vi "WPI_SimpleGyro_Loop.vi"(8 "error in":errorcluster, 11 "SimpleGyroDevRef":T1) -> (0 "error out":errorcluster)   [LabVIEW 2014, in "SimpleGyro.lvlib"]
doc: "Periodically reads the SimpleGyro and makes data available to your robot project. Place this block within PeriodicTasks.vi."
uses:
  SimpleGyro.lvlib
  WPI_SimpleGyroDevRef.ctl
  <vilib>/Rock Robotics/SystemInterfaces/Typedef/FPGA_TypedefDigitalModule.ctl
  <vilib>/Rock Robotics/SystemInterfaces/spilib/spi_bus.ctl
  <vilib>/Rock Robotics/WPI/SPI/WPI_SPIDevRef.ctl
  <vilib>/Platform/TimedLoop/XDataNode/timing_clust.ctl
  <vilib>/Platform/TimedLoop/XDataNode/nitl_modes.ctl
  <vilib>/Platform/TimedLoop/XDataNode/wakeup.ctl
  <vilib>/platform/TimedLoop/XDataNode/XDataNode.xnode
  <vilib>/Platform/TimedLoop/XDataNode/XDNodeRunTimeDep.lvlib
  <vilib>/ptbypt/NI_PtbyPt.lvlib
panel:
  out "mean":dbl format="%0.2f"
  in  "Calibrate":bool
  out "Angle":dbl
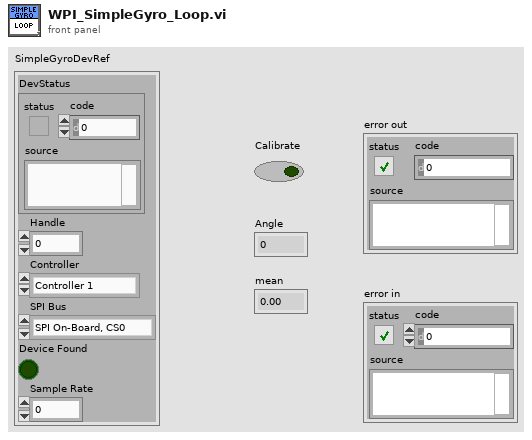
[diagram p1: front panel]
types:
  T1 = typedef "SimpleGyro.lvlib/WPI_SimpleGyroDevRef.ctl" = cluster{"DevStatus":errorcluster, "Handle":i32, "Controller":T2, "SPI Bus":T3, "Device Found":bool, "Sample Rate":dbl}
  T2 = typedef "FPGA_TypedefDigitalModule.ctl" = enum16{"Controller 1"}
  T3 = typedef "spi_bus.ctl" = enum16{"SPI On-Board, CS0", "SPI On-Board, CS1", "SPI On-Board, CS2", "SPI On-Board, CS3", "SPI MXP", "Invalid"}
  T4 = typedef "WPI_SPIDevRef.ctl" = cluster{"DevStatus":errorcluster, "Handle":i32, "Controller":T2, "SPI Bus":T3}
  T5 = typedef "XDNodeRunTimeDep.lvlib/timing_clust.ctl" = cluster{"Expected End [f-1]":u64, "Actual End [f-1]":u64, "Finished Late? [f-1]":bool, "Expected End [i-1]":u64, "Actual End [i-1]":u64, "Finished Late? [i-1]":bool, "Expected Start [i]":u64, "Actual Start [i]":u64, "Expected Start [f]":u64, "Actual Start [f]":u64, "Source Name":string, "Structure Name":string, "Period":i64, "Deadline":i64, "Offset":i64, "Start":i64, "Priority":i32, "Timeout":i32, "Mode":T6, "Wakeup Reason":T7, "Error":errorcluster, "Source Type":string, "Secondary Source Type":string, "Global End Time":u64, "Global Start Time":u64, "Frame Duration":u64, "Iteration Duration":u64, "Assigned CPU":i32, "I/O Scan Engine Mode":u32}
  T6 = typedef "XDNodeRunTimeDep.lvlib/nitl_modes.ctl" = enum32{"No Change", "Process missed periods, maintain original phase", "Discard missed periods, maintain original phase", "Process missed periods, ignore original phase", "Discard missed periods, ignore original phase"}
  T7 = typedef "XDNodeRunTimeDep.lvlib/wakeup.ctl" = enum32{"Normal", "Aborted", "Asynchronous wakeup", "Timing source error", "Timed loop error", "Timeout"}
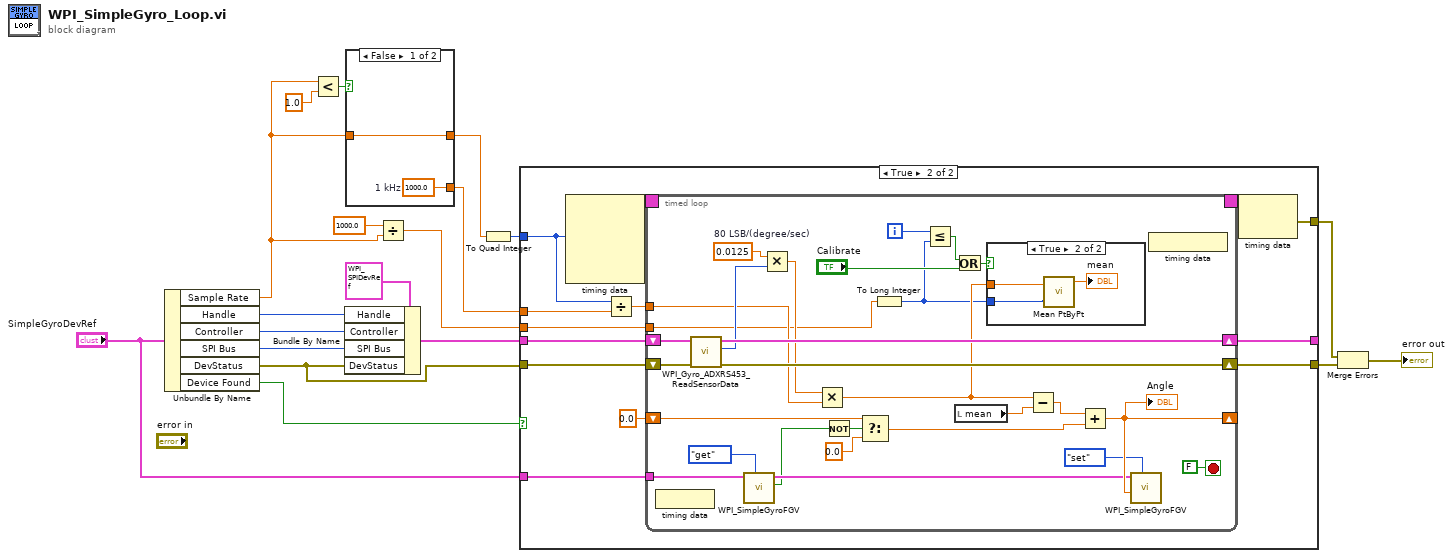
[diagram p0: block diagram]
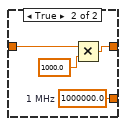
[diagram p2: hidden frame]
diagram:
  n1 = Unbundle By Name("SimpleGyroDevRef") -> ("Sample Rate"=w2:dbl, "Handle"=w18:i32, "Controller"=w17:T2, "SPI Bus"=w16:T3, "DevStatus"=w14:errorcluster, "Device Found"=w13:bool)
  n2 = Less?(x=w2, y=1.0) -> (x < y?=w4:bool)
  n3 = Bundle By Name(cluster=T4 {"DevStatus"={"status"=FALSE, "code"=0, "source"=""}, "Handle"=0, "Controller"=enum."Controller 1", "SPI Bus"=enum."Invalid"} ("SPIDevRef out"), "Handle"=w18, "Controller"=w17, "SPI Bus"=w16, "DevStatus"=w14) -> (w15:T4)
  n4 = case shown="False" w4 {
    tunnel: w2 -> [w21 w25]
    tunnel: [w21 w24] -> w11
    tunnel: [w20 w22] -> w9
    frame False {
      w20 = 1000.0  # 1 kHz
    }
    frame True {
      w22 = 1000000.0  # 1 MHz
      n5 = Multiply(x=w25, y=1000.0) -> (x*y=w24:dbl)
    }
  }
  n6 = Divide(x=1000.0 ("y"), y=w2) -> (x/y=w1:dbl)
  n7 = To Quad Integer(1:w11) -> (0:w10:i64)
  n8 = case shown="True" w13 {
    tunnel: w15 -> [w27 w38]
    tunnel: w14 -> [w26 w37]
    tunnel: [w26 w36] -> w7
    tunnel: [w27 w35] -> _
    tunnel: w10 -> [_ w33]
    tunnel: w9 -> [_ w32]
    tunnel: "SimpleGyroDevRef" -> [_ w31]
    tunnel: [_ w30] -> w6
    tunnel: w1 -> [_ w28]
    frame False {
    }
    frame True {
      n9 = node-c288(w33) -> (w40:T5)  [unwired: 3 in]
      n10 = Divide(x=w33, y=w32) -> (x/y=w34:dbl)
      n11 = timed-loop {
        shift-right: [w66] -> w35
        shift-left: w38 -> [w68]
        shift-right: [w62] -> w36
        shift-left: w37 -> [w67]
        timing: w40 -> [_]
        timing-out: [_] -> w39
        shift-right: [w47] -> _
        shift-left: 0.0 -> [w63]
        tunnel: w34 -> [w43]
        tunnel: w31 -> [w49]
        tunnel: w28 -> [w41]
        i -> [w52]
        stop <- FALSE stop-if-true
        w64 = 0.0125  # 80 LSB/(degree/sec)
        n12 = node-c288() -> ()  [unwired: 1 in]
        n13 = call <vilib>:"WPI_Gyro_ADXRS453_ReadSensorData.vi"("error in (no error)"=w67, "SPIDevRef in"=w68) -> ("error out"=w62:errorcluster, "Sensor Data (n-1)"=w65:i16, "SPIDevRef out"=w66:T4)  [unwired: 5 in, 2 out]
        n14 = call "WPI_SimpleGyroFGV.vi"("Operation"=enum16{"set", "get"}."get", "SimpleGyroDevRef"=w49) -> ("Reset?"=w44:bool, "SimpleGyroDevRef"=w45:T1)  [unwired: 7 in, 1 out]
        n15 = Multiply(x=w64, y=w65) -> (x*y=w59:dbl)
        n16 = Multiply(x=w59, y=w43) -> (x*y=w58:dbl)
        n17 = Not(x=w44) -> (.not. x?=w50:bool)
        n18 = Select(t=w63, s=w50, f=0.0 ("t")) -> (s? t:f=w56:dbl)
        n19 = To Long Integer(number=w41) -> (32bit integer=w42:i32)
        n20 = Less Or Equal?(x=w52, y=w42) -> (x <= y?=w51:bool)
        n21 = Or(x=w51, y="Calibrate") -> (x .or. y?=w53:bool)
        n22 = local read "mean"() -> (w54:dbl)
        n23 = case shown="True" w53 {
          tunnel: w58 -> [_ w70]
          tunnel: w42 -> [_ w69]
          frame False {
          }
          frame True {
            n24 = call <vilib>:"Mean PtByPt.vi"("x"=w70, "sample length"=w69) -> ("mean"=→"mean":dbl)  [unwired: 2 in, 1 out]
          }
        }
        n25 = Subtract(x=w58, y=w54) -> (x-y=w61:dbl)
        n26 = Add(x=w61, y=w56) -> (x+y=w47:dbl)
        "Angle" <- w47
        n27 = call "WPI_SimpleGyroFGV.vi"("Operation"=enum16{"set", "get"}."set", "Angle"=w47, "SimpleGyroDevRef"=w45) -> ()  [unwired: 6 in, 3 out]
        n28 = node-c288() -> ()  [unwired: 1 out]
      }
      n29 = node-c288(w39) -> (w30:errorcluster)
    }
  }
  n30 = Merge Errors(w6, w7) -> (→"error out":errorcluster)
